vi "Climb Globals.vi"() -> ()   [LabVIEW 2016]
uses:
  Climb Notifier.ctl
  Climb Control Type.ctl
panel:
  in  "Left Climb Motor":string="Left Climb Motor"
  in  "Right Climb Motor":string="Right Climb Motor"
  in  "Climb DVR":refnum<data-value>
  in  "Climb Notifier":refnum<notifier>
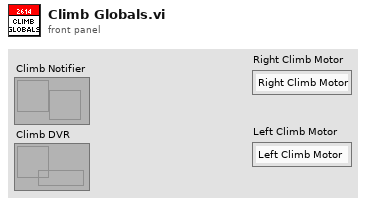
[diagram p1: front panel]
diagram:
